vi "Write Always Repeat First Node.vi"(8 "error in (no error)":errorcluster, 10 "Always Repeat First Node":bool, 11 "Parallel_Interleaved in":refnum<class "Parallel_Interleaved.lvclass">) -> (0 "error out":errorcluster, 3 "Parallel_Interleaved out":refnum<class "Parallel_Interleaved.lvclass">)   [LabVIEW 2021, in "BT.lvlib" / "Parallel_Interleaved.lvclass"]
uses:
  Parallel_Interleaved.lvclass
  Parallel_Interleaved.lvclass/Parallel_Interleaved.ctl
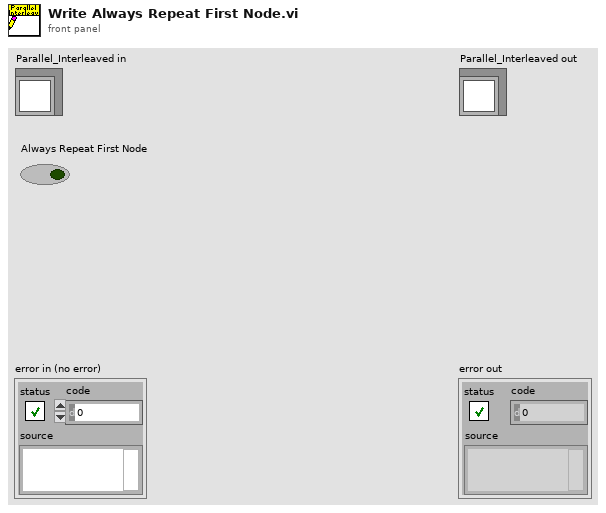
[diagram p1: front panel]
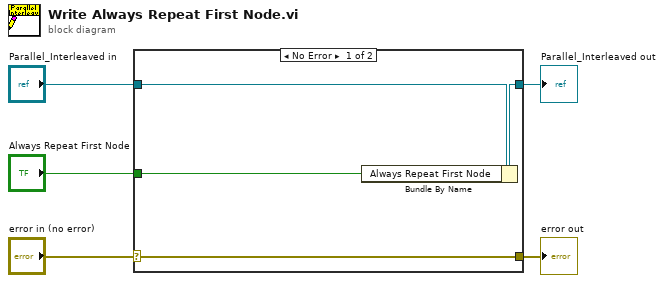
[diagram p0: block diagram]
diagram:
  n1 = case shown="No Error" "error in (no error)" {
    selector: "error in (no error)" -> [w9 w10]
    tunnel: [w9 w10] -> w4
    tunnel: [w7 w11] -> w2
    tunnel: "Parallel_Interleaved in" -> [w8 w11]
    tunnel: "Always Repeat First Node" -> [w6 _]
    frame No Error {
      n2 = Bundle By Name(cluster=w8, "Always Repeat First Node"=w6) -> (w7:refnum<class "Parallel_Interleaved.lvclass">)
    }
    frame Error {
    }
  }
  "error out" <- w4
  "Parallel_Interleaved out" <- w2
